vi "CF_TC to PGSQL.vi"(8 "error in (no error)":errorcluster, 9 "calibration string":string, 10 "description string":string, 11 "dbl":dbl[](array[numeric])) -> (0 "error out":errorcluster)   [LabVIEW 2016]
panel:
  # "CF TC to PGSQL"
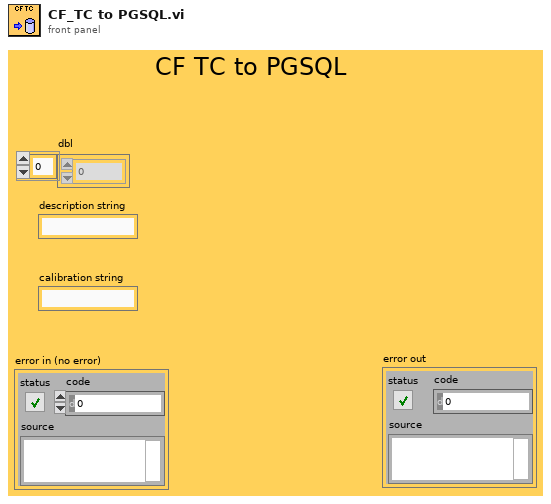
[diagram p1: front panel]
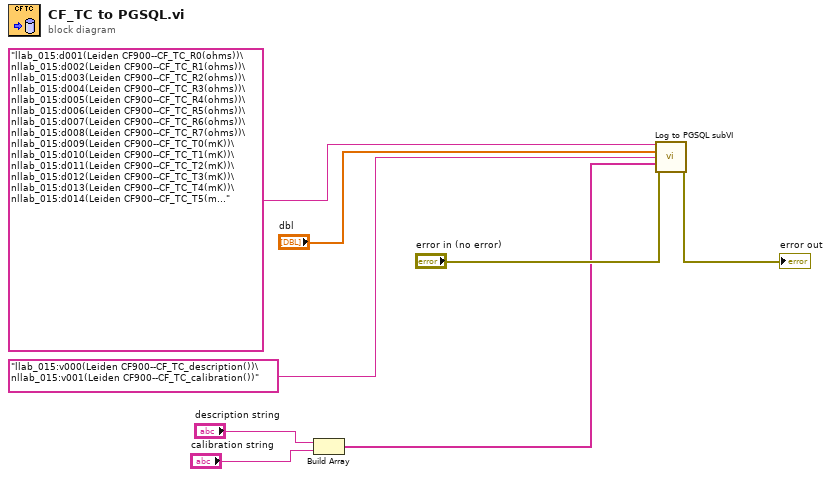
[diagram p0: block diagram]
diagram:
  n1 = Build Array("description string", "calibration string") -> (w3:string[])
  n2 = call "Log to PGSQL subVI.vi"("dbl paths"="llab_015:d001(Leiden CF900--CF_TC_R0(ohms))\nllab_015:d002(Leiden CF900--CF_TC_R1(ohms))\nllab_015:d003(Leiden CF900--CF_TC_R2(ohms))\nllab_015:d004(Leiden CF900--CF_TC_R3(ohms))\nllab_015:d005(Leiden CF900--CF_TC_R4(ohms))\nllab_015:d006(Leiden CF900--CF_TC_R5(ohms))\nllab_015:d007(Leiden CF900--CF_TC_R6(ohms))\nllab_015:d008(Leiden CF900--CF_TC_R7(ohms))\nllab_015:d009(Leiden CF900--CF_TC_T0(mK))\nllab_015:d010(Leiden CF900--CF_TC_T1(mK))\nllab_015:d011(Leiden CF900--CF_TC_T2(mK))\nllab_015:d012(Leiden CF900--CF_TC_T3(mK))\nllab_015:d013(Leiden CF900--CF_TC_T4(mK))\nllab_015:d014(Leiden CF900--CF_TC_T5(mK))\nllab_015:d015(Leiden CF900--CF_TC_T6(mK))\nllab_015:d016(Leiden CF900--CF_TC_T7(mK))\nllab_015:d017(Leiden CF900--CF_TC_I0(Amp))\nllab_015:d018(Leiden CF900--CF_TC_I1(Amp))\nllab_015:d019(Leiden CF900--CF_TC_I2(Amp))\nllab_015:d020(Leiden CF900--CF_TC_I3(Amp))", "dbl []"="dbl", "string paths"="llab_015:v000(Leiden CF900--CF_TC_description())\nllab_015:v001(Leiden CF900--CF_TC_calibration())", "string []"=w3, "error in (no error)"="error in (no error)") -> ("error out"=→"error out":errorcluster)  [unwired: 10 in]
